vi "Day 21-Part 1.vi"() -> ()   [LabVIEW 2021]
uses:
  Day 21-Turn Cluster.ctl
  Day 21-Player Turn.ctl
panel:
  out "Dice Roll Count":u64
  out "Player 2 Score":u64
  out "Player 1 Score":u64
  in  "Player 2 Starting Position":u64=3
  in  "Player 1 Starting Position":u64=10
  out "Solution":u64
  # "Example:\nPlayer 1 starting position: 4\nPlayer 2 starting position: 8"
  # "Input:\nPlayer 1 starting position: 10\nPlayer 2 starting position: 3"
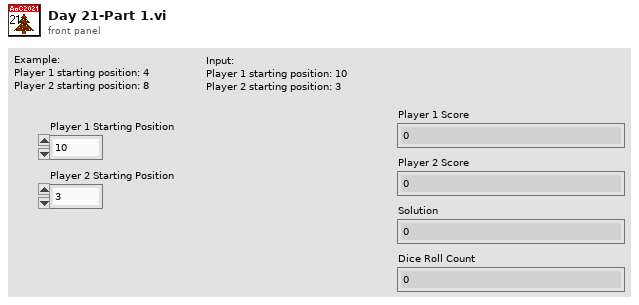
[diagram p1: front panel]
types:
  T1 = typedef "Day 21-Turn Cluster.ctl" = cluster{"Player 1 Position":u64, "Player 1 Score":u64, "Player 2 Position":u64, "Player 2 Score":u64, "Player Turn":T2}
  T2 = typedef "Day 21-Player Turn.ctl" = enum16{"Player 1", "Player 2"}
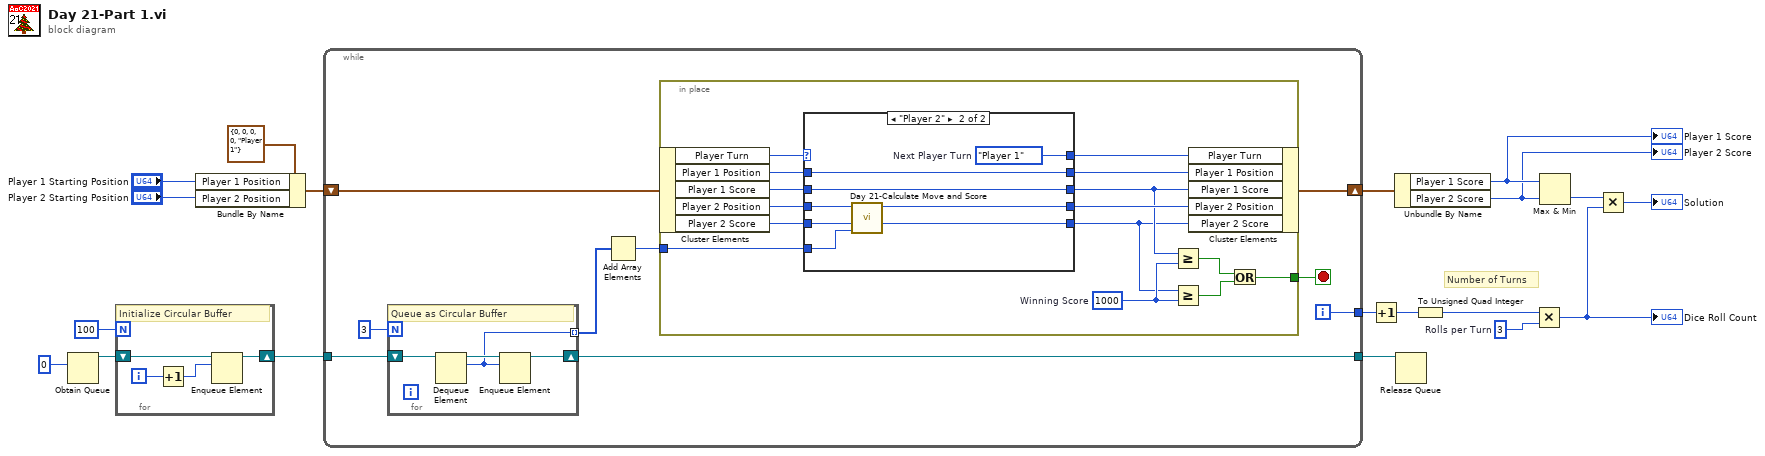
[diagram p0: block diagram]
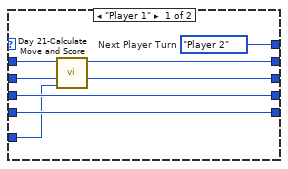
[diagram p2: hidden frame]
diagram:
  w4 = u64 3  # Rolls per Turn
  # "Number of Turns"
  n1 = Obtain Queue(element data type=u64 0) -> (queue out=w9:refnum<queue>)  [unwired: 4 in, 2 out]
  n2 = for {
    N: 100 -> [_]
    shift-right: [w20] -> w7
    shift-left: w9 -> [w23]
    i -> [w22]
    # "Initialize Circular Buffer"
    n3 = Increment(x=w22) -> (x+1=w21:i32)
    n4 = Enqueue Element(queue=w23, element=w21) -> (queue out=w20:refnum<queue>)  [unwired: 2 in, 2 out]
  }
  n5 = Bundle By Name(cluster=T1 {"Player 1 Position"=0, "Player 1 Score"=0, "Player 2 Position"=0, "Player 2 Score"=0, "Player Turn"=enum."Player 1"} ("State"), "Player 1 Position"="Player 1 Starting Position", "Player 2 Position"="Player 2 Starting Position") -> (w16:T1)
  n6 = while {
    shift-right: [w30] -> w15
    shift-left: w16 -> [w32]
    tunnel: w7 -> [w27]
    tunnel: [w26] -> w6
    tunnel: [w24] -> w5
    i -> [w24]
    stop <- w29 stop-if-true
    n7 = for {
      N: 3 -> [_]
      tunnel: [w34] -> w25 mode=indexing
      shift-right: [w33] -> w26
      shift-left: w27 -> [w36]
      # "Queue as Circular Buffer"
      n8 = Dequeue Element(queue=w36) -> (queue out=w35:refnum<queue>, element=w34:u64)  [unwired: 2 in, 2 out]
      n9 = Enqueue Element(queue=w35, element=w34) -> (queue out=w33:refnum<queue>)  [unwired: 2 in, 2 out]
    }
    n10 = Add Array Elements(numeric array=w25) -> (sum=w31:u64)
    n11 = in-place {
      in-place-border: [w43] -> w29
      in-place-border: w31 -> [w37]
      w44 = u64 1000  # Winning Score
      n12 = in-place-cluster #1(w32) -> ("Player Turn"=w51:T2, "Player 1 Position"=w50:u64, "Player 1 Score"=w49:u64, "Player 2 Position"=w47:u64, "Player 2 Score"=w45:u64)
      n13 = case shown="\"Player 2\"" w51 {
        tunnel: w50 -> [w59 w61]
        tunnel: w47 -> [w58 w66]
        tunnel: w37 -> [w54 w62]
        tunnel: w49 -> [w53 w60]
        tunnel: [w52 w60] -> w39
        tunnel: [w56 w61] -> w48
        tunnel: [w58 w65] -> w46
        tunnel: [w57 w63] -> w38
        tunnel: w45 -> [w57 w64]
        tunnel: [w55 w67] -> w42
        frame "Player 1" {
          w55 = Day_21-Player_Turn."Player 2"  # Next Player Turn
          n14 = call "Day 21-Calculate Move and Score.vi"("Dice Roll Sum"=w54, "Score in"=w53, "Position in"=w59) -> ("Score out"=w52:u64, "Position out"=w56:u64)  [unwired: 7 in]
        }
        frame "Player 2" {
          w67 = Day_21-Player_Turn."Player 1"  # Next Player Turn
          n15 = call "Day 21-Calculate Move and Score.vi"("Dice Roll Sum"=w62, "Score in"=w64, "Position in"=w66) -> ("Score out"=w63:u64, "Position out"=w65:u64)  [unwired: 7 in]
        }
      }
      n16 = Greater Or Equal?(x=w39, y=w44) -> (x >= y?=w41:bool)
      n17 = Greater Or Equal?(x=w38, y=w44) -> (x >= y?=w40:bool)
      n18 = in-place-cluster #1("Player Turn"=w42, "Player 1 Position"=w48, "Player 1 Score"=w39, "Player 2 Position"=w46, "Player 2 Score"=w38) -> (w30:T1)
      n19 = Or(x=w41, y=w40) -> (x .or. y?=w43:bool)
    }
  }
  n20 = Increment(x=w5) -> (x+1=w1:i32)
  n21 = Unbundle By Name(w15) -> ("Player 1 Score"=w14:u64, "Player 2 Score"=w13:u64)
  "Player 1 Score" <- w14
  "Player 2 Score" <- w13
  n22 = Release Queue(queue=w6) -> ()  [unwired: 2 in, 3 out]
  n23 = To Unsigned Quad Integer(1:w1) -> (0:w2:u64)
  n24 = Multiply(x=w2, y=w4) -> (x*y=w3:u64)
  "Dice Roll Count" <- w3
  n25 = Max & Min(x=w14, y=w13) -> (min(x,y)=w12:u64)  [unwired: 1 out]
  n26 = Multiply(x=w12, y=w3) -> (x*y=→"Solution":u64)
